vi "set_motion_default_speed.vi"(8 "error in (no error)":errorcluster caption="错误输入（无错误）", 10 "default speed":i32, 11 "OneMotion 输入":refnum<class "OneMotion.lvclass">) -> (0 "error out":errorcluster caption="错误输出", 3 "OneMotion 输出":refnum<class "OneMotion.lvclass">)   [LabVIEW 2016, in "MotionControl.lvlib" / "OneMotion.lvclass"]
uses:
  <userlib>/MotionControl/OneMotion/OneMotion.lvclass
  <userlib>/MotionControl/OneMotion/OneMotion.lvclass/OneMotion.ctl
  <userlib>/MotionControl/StepMotor/StepMotor.lvclass/StepMotor.ctl
  <userlib>/MotionControl/StepMotor/StepMotor.lvclass
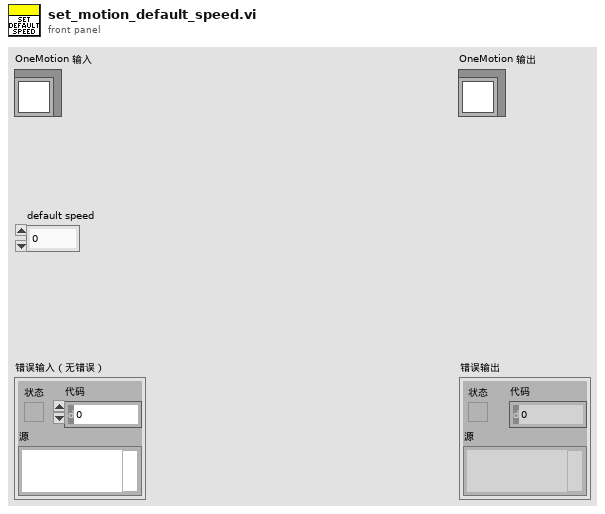
[diagram p1: front panel]
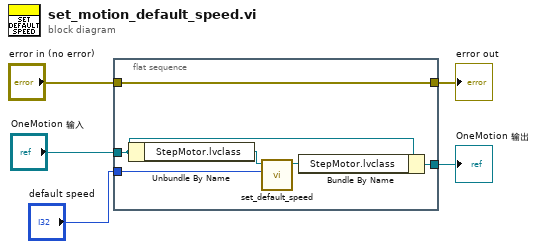
[diagram p0: block diagram]
diagram:
  n1 = flat-sequence {
    tunnel: [w11] -> w5
    tunnel: [w6] -> w3
    tunnel: "OneMotion 输入" -> [w8]
    tunnel: "error in (no error)" -> [w11]
    tunnel: "default speed" -> [w10]
    frame #0 {
      n2 = Unbundle By Name(w8) -> ("StepMotor.lvclass"=w9:refnum<class "StepMotor.lvclass">)
      n3 = call <userlib>:"set_default_speed.vi"("expected speed"=w10, "StepMotor输入"=w9) -> ("StepMotor输出"=w7:refnum<class "StepMotor.lvclass">)  [unwired: 8 in, 1 out]
      n4 = Bundle By Name(cluster=w8, "StepMotor.lvclass"=w7) -> (w6:refnum<class "OneMotion.lvclass">)
    }
  }
  "error out" <- w5
  "OneMotion 输出" <- w3
